vi "AvrLines.vi"(0 "slope (m)":dbl[][](array[numeric]) format="%.2f", 1 "Avg #":i32=10, 2 "intercept (b) in":dbl[][](array[numeric]) format="%.2f", 3 "midband fit in":dbl[][](array[numeric]) format="%.2f") -> (4 "start index AVG":dbl, 5 "slope avr":dbl[](array[numeric]) format="%.2f", 6 "intercept avr":dbl[](array[numeric]) format="%.2f", 7 "midband avr":dbl[](array[numeric]) format="%.2f")   [LabVIEW 2022 SP3]
uses:
  <vilib>/Analysis/baseanly.llb/Mean (DBL).vi
  <vilib>/Analysis/NI_AALBase.lvlib
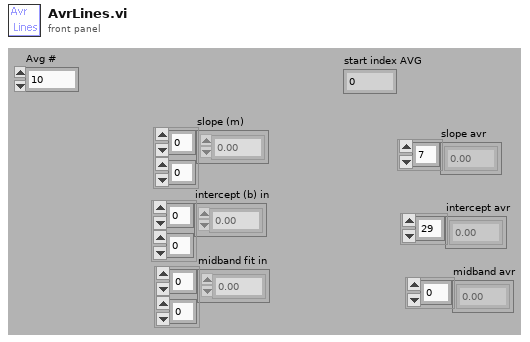
[diagram p1: front panel]
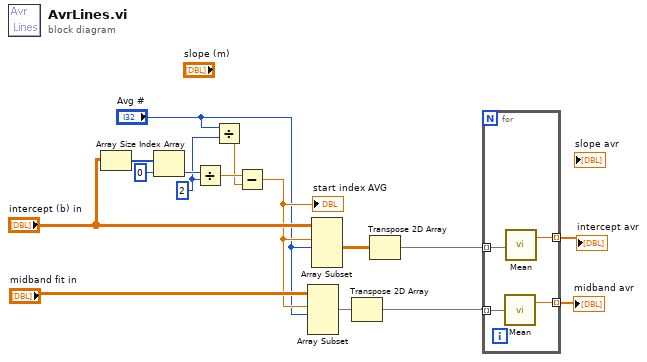
[diagram p0: block diagram]
diagram:
  w11 = 2
  n1 = Array Size(array="intercept (b) in") -> (size(s)=w16:i32[])
  n2 = Index Array(array=w16, index=0) -> (element=w14:i32)
  n3 = Divide(x=w14, y=w11) -> (x/y=w12:dbl)
  n4 = Divide(x="Avg #", y=w11) -> (x/y=w10:dbl)
  n5 = Subtract(x=w12, y=w10) -> (x-y=w4:dbl)
  "start index AVG" <- w4
  n6 = Array Subset(array="midband fit in", index (row)=w4, length (row)="Avg #") -> (w8:dbl[][])  [unwired: 2 in]
  n7 = Array Subset(array="intercept (b) in", index (row)=w4, length (row)="Avg #") -> (w7:dbl[][])  [unwired: 2 in]
  n8 = Transpose 2D Array(2D array=w8) -> (transposed array=w2:dbl[][])
  n9 = Transpose 2D Array(2D array=w7) -> (transposed array=w3:dbl[][])
  n10 = for {
    tunnel: w2 -> [w20] mode=indexing
    tunnel: w3 -> [w19] mode=indexing
    tunnel: [w18] -> w6 mode=indexing
    tunnel: [w17] -> w9 mode=indexing
    n11 = call-poly <vilib>:"Mean.vi"("X"=w20) -> ("mean"=w17:dbl)  [unwired: 1 out]
    n12 = call-poly <vilib>:"Mean.vi"("X"=w19) -> ("mean"=w18:dbl)  [unwired: 1 out]
  }
  "intercept avr" <- w6
  "midband avr" <- w9
